vi "area ROI.vi"(8 "error in":errorcluster, 9 "ROI max":dbl, 10 "ROI min":dbl, 11 "Sum Spectrum":cluster{"Ramp Pattern":dbl[], "Array":i32[]}[](graph)) -> (0 "error out":errorcluster, 2 "ROI Area":cluster{"Array":dbl[], "Array":i32[]}, 3 "XY Graph":cluster{"Channel":dbl[], "Intensity":i32[]}[](graph))   [LabVIEW 2023]
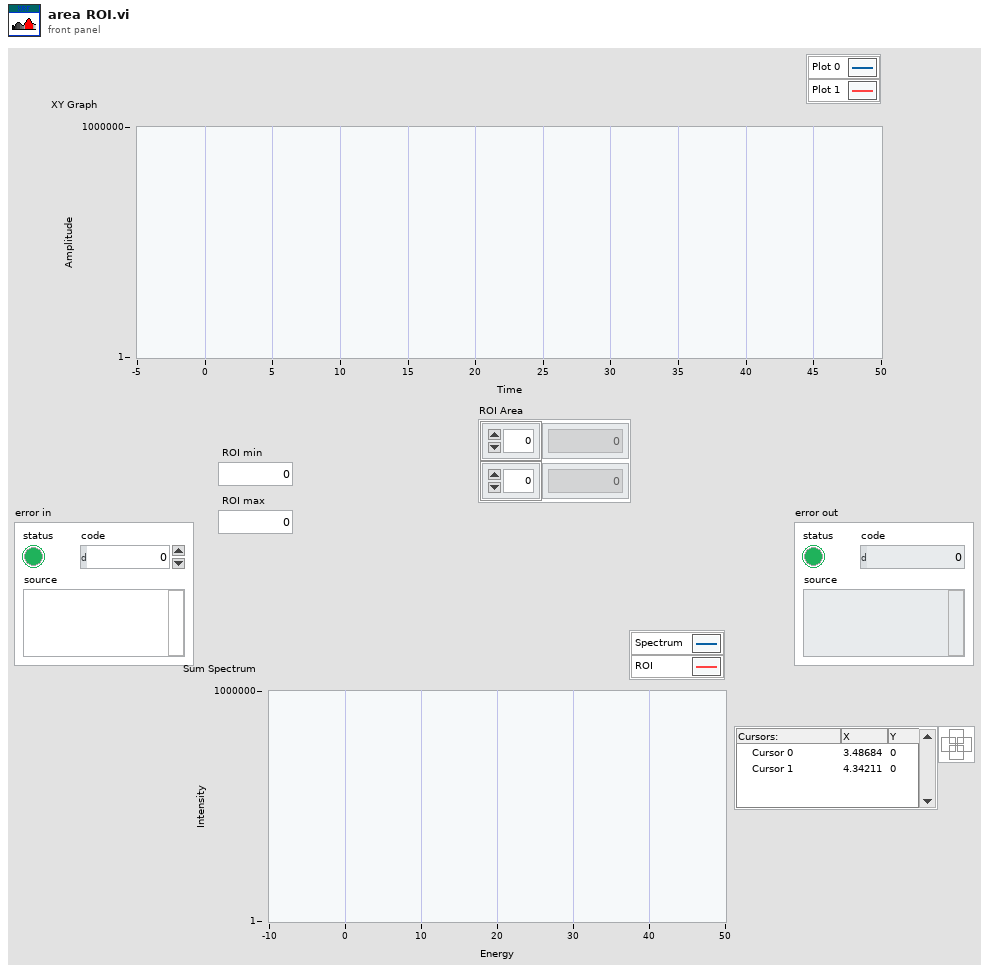
[diagram p1: front panel]
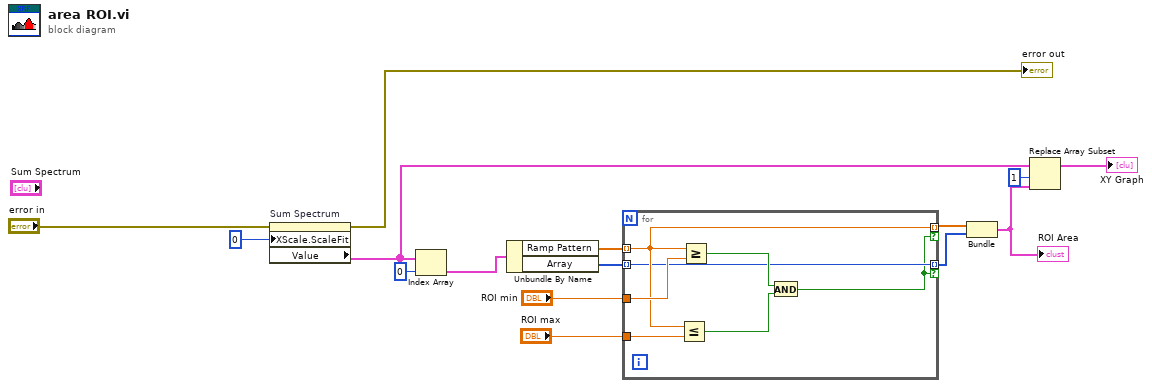
[diagram p0: block diagram]
diagram:
  n1 = property on="Sum Spectrum" class="XYGraph (strict)"(error in="error in", "XScale.ScaleFit"=u8 0 ("Y Scale.Scale Fit")) -> (error out=→"error out":errorcluster, "Value"=w4:cluster{"Ramp Pattern":dbl[], "Array":i32[]}[])  [unwired: 1 in, 1 out]
  n2 = Index Array(array=w4, index=0) -> (element=w5:cluster{"Ramp Pattern":dbl[], "Array":i32[]})
  n3 = Unbundle By Name(w5) -> ("Ramp Pattern"=w13:dbl[], "Array"=w12:i32[])
  n4 = for {
    tunnel: w13 -> [w18] mode=indexing
    tunnel: w12 -> [w17] mode=indexing
    tunnel: "ROI min" -> [w22]
    tunnel: "ROI max" -> [w21]
    tunnel: [w18] -> w9 mode=indexing if=w16
    tunnel: [w17] -> w8 mode=indexing if=w16
    n5 = Less Or Equal?(x=w18, y=w21) -> (x <= y?=w19:bool)
    n6 = Greater Or Equal?(x=w18, y=w22) -> (x >= y?=w20:bool)
    n7 = And(x=w20, y=w19) -> (x .and. y?=w16:bool)
  }
  n8 = Bundle(w9, w8) -> (w2:cluster{dbl[], i32[]})  [unwired: 1 in]
  "ROI Area" <- w2
  n9 = Replace Array Subset(array=w4, new element=w2, index=1) -> (→"XY Graph":cluster{"Ramp Pattern":dbl[], "Array":i32[]}[])
